vi "Simple Reader.vi"(8 "error in (no error)":errorcluster, 11 "Signal Recovery Driver in":refnum<class "Signal Recovery Driver.lvclass">) -> (0 "error out":errorcluster, 2 "Signals":dbl[](array[numeric]), 3 "Signal Recovery Driver out":refnum<class "Signal Recovery Driver.lvclass">)   [LabVIEW 2025, in "Signal Recovery Driver.lvclass"]
uses:
  Signal Recovery Driver.lvclass
  C:/GitHub/NHMFL_Core/Libraries/Instruments/VISA Instrument/VISA Instrument.lvclass
  VISA Instrument/VISA Instrument.lvclass/VISA Instrument.ctl
  VISA Instrument/Read VISA resource.vi
  VISA Instrument/Write VISA resource.vi
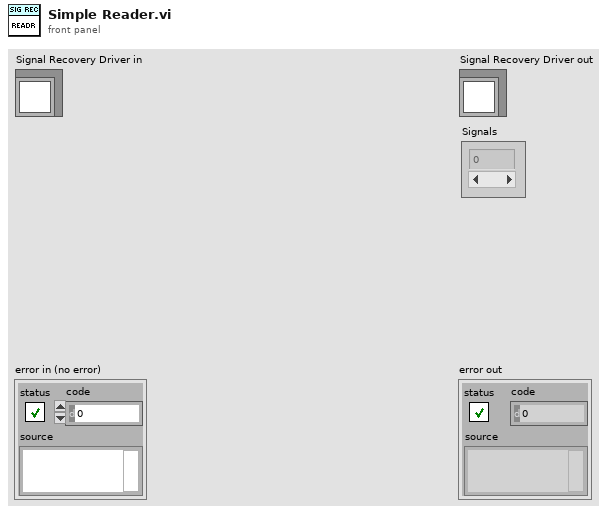
[diagram p1: front panel]
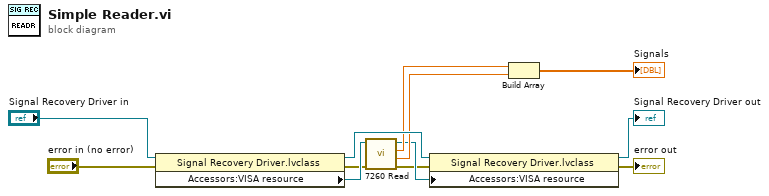
[diagram p0: block diagram]
diagram:
  n1 = property class="Signal Recovery Driver.lvclass"(reference="Signal Recovery Driver in", error in="error in (no error)") -> (reference out=w12:refnum<class "Signal Recovery Driver.lvclass">, error out=w7:errorcluster, "Accessors:VISA resource"=w11:refnum<visa-resource-name>)
  n2 = call "7260 Read.vi"("error in (no error)"=w7, "VISA Resource Name"=w11) -> ("error out"=w6:errorcluster, "Y"=w9:dbl, "X"=w10:dbl, "VISA Resource Name Out"=w8:refnum<visa-resource-name>)  [unwired: 5 in, 1 out]
  n3 = property class="Signal Recovery Driver.lvclass"(reference=w12, error in=w6, "Accessors:VISA resource"=w8) -> (reference out=→"Signal Recovery Driver out":refnum<class "Signal Recovery Driver.lvclass">, error out=→"error out":errorcluster)
  n4 = Build Array(w10, w9) -> (→"Signals":dbl[])
